vi "TimeoutTask.vi"(0 "AbortQueue":refnum<queue>, 1 "TimeoutID":u32, 2 "TimeoutName":string, 3 "TimeoutInterface":refnum<class "ITimerTimeout.lvclass">, 4 "TimeoutTime(s)":dbl, 5 "error in (no error)":errorcluster) -> (19 "error out":errorcluster)   [LabVIEW 2020, in "LcTimer.lvclass"]
uses:
  LcTimer.lvclass
  ITimerTimeout_Interface/ITimerTimeout.lvclass
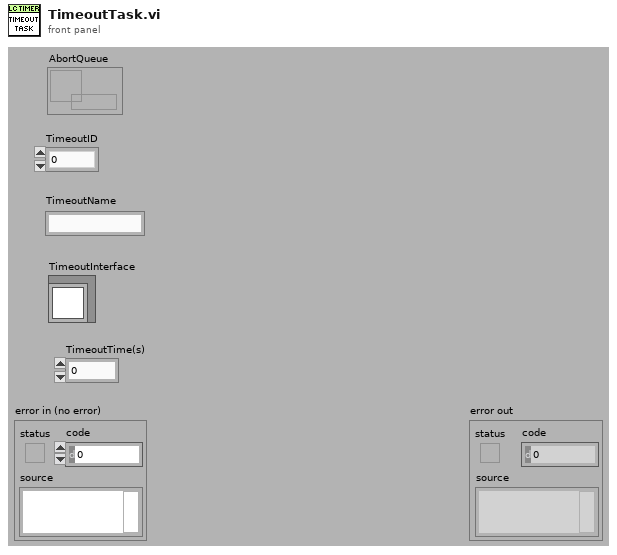
[diagram p1: front panel]
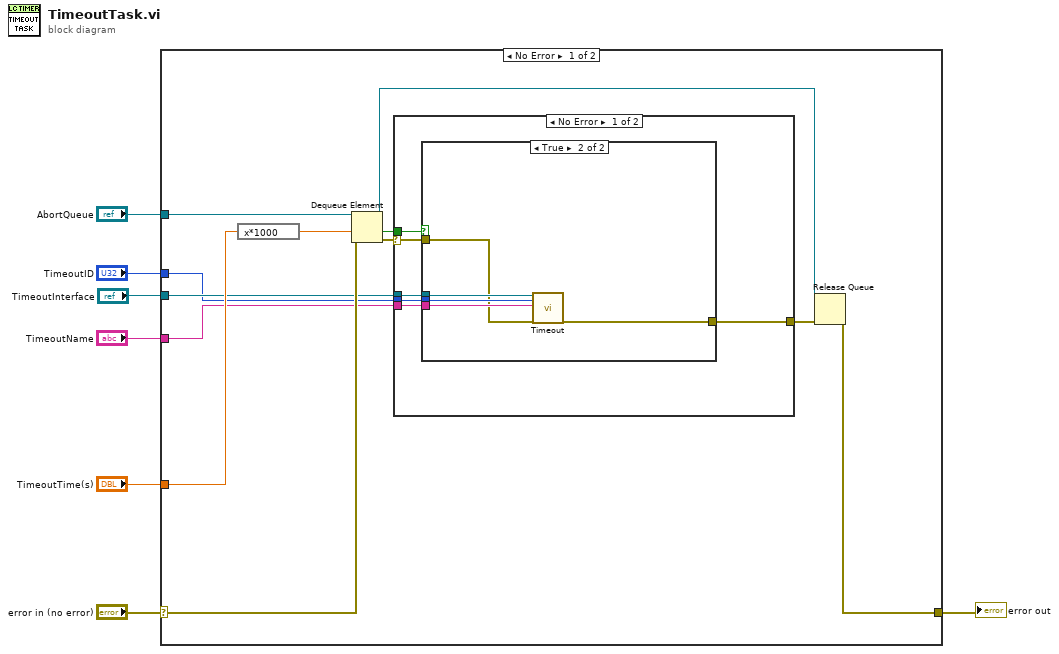
[diagram p0: block diagram]
diagram:
  n1 = case shown="No Error" "error in (no error)" {
    selector: "error in (no error)" -> [w16 w33]
    tunnel: [w8 w33] -> w6
    tunnel: "AbortQueue" -> [w19 _]
    tunnel: "TimeoutTime(s)" -> [w18 _]
    tunnel: "TimeoutInterface" -> [w13 _]
    tunnel: "TimeoutID" -> [w12 _]
    tunnel: "TimeoutName" -> [w11 _]
    frame No Error {
      n2 = expression code="x*1000"(w18) -> (w17:dbl)
      n3 = Dequeue Element(queue=w19, timeout in ms (-1)=w17, error in (no error)=w16) -> (queue out=w10:refnum<queue>, timed out?=w15:bool, error out=w14:errorcluster)  [unwired: 1 out]
      n4 = case shown="No Error" w14 {
        selector: w14 -> [w21 w32]
        tunnel: w15 -> [w25 _]
        tunnel: w13 -> [w24 _]
        tunnel: w12 -> [w23 _]
        tunnel: w11 -> [w22 _]
        tunnel: [w20 w32] -> w9
        frame No Error {
          n5 = case shown="True" w25 {
            tunnel: w24 -> [_ w31]
            tunnel: w23 -> [_ w30]
            tunnel: w22 -> [_ w29]
            tunnel: w21 -> [w26 w28]
            tunnel: [w26 w27] -> w20
            frame False {
            }
            frame True {
              n6 = call-dynamic "Timeout.vi"("Interface In"=w31, "TimeoutID"=w30, "TimeoutName"=w29, "error in (no error)"=w28) -> ("error out"=w27:errorcluster)  [unwired: 14 in, 1 out]
            }
          }
        }
        frame Error {
        }
      }
      n7 = Release Queue(queue=w10, error in (no error)=w9) -> (error out=w8:errorcluster)  [unwired: 1 in, 2 out]
    }
    frame Error {
    }
  }
  "error out" <- w6
